vi "open camera settings.vi"(8 "error in (no error)":errorcluster, 11 "Camera Tester in":refnum<class "Camera Tester.lvclass">) -> (0 "error out":errorcluster, 3 "Camera Tester out":refnum<class "Camera Tester.lvclass">)   [LabVIEW 2014, in "Camera Tester.lvlib" / "Camera Tester.lvclass"]
uses:
  Camera Tester.lvclass
  Camera Tester.lvclass/Camera Tester.ctl
  <vilib>/ActorFramework/Message Enqueuer/Message Enqueuer.lvclass/Message Enqueuer.ctl
  <vilib>/ActorFramework/Message Enqueuer/Enqueue.vi
  <vilib>/ActorFramework/Message Priority Queue/Priority Enqueue.vi
  Camera Actor/Camera Actor Messages/open camera settings Msg/open camera settings Msg.lvclass
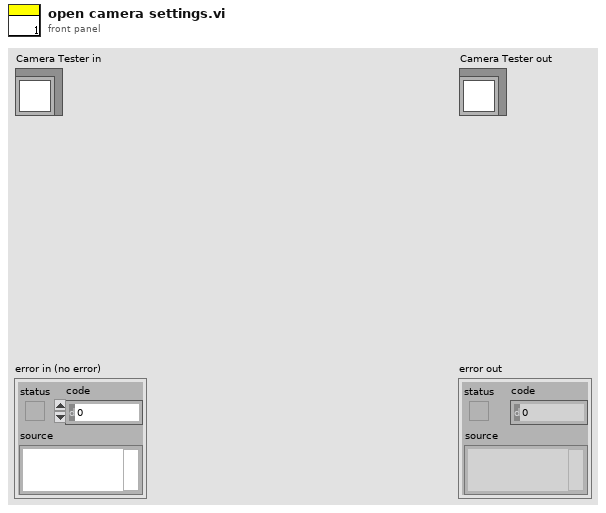
[diagram p1: front panel]
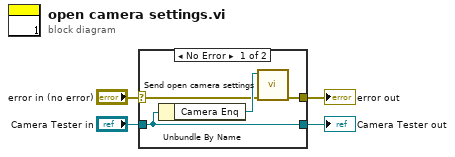
[diagram p0: block diagram]
diagram:
  n1 = case shown="No Error" "error in (no error)" {
    selector: "error in (no error)" -> [w6 w10]
    tunnel: [w5 w10] -> w3
    tunnel: [w8 w9] -> w1
    tunnel: "Camera Tester in" -> [w8 w9]
    frame No Error {
      n2 = Unbundle By Name(w8) -> ("Camera Enq"=w7:refnum<class "Message Enqueuer.lvclass">)
      n3 = call "Send open camera settings.vi"("error in (no error)"=w6, "Message Enqueuer"=w7) -> ("error out"=w5:errorcluster)  [unwired: 8 in, 1 out]
    }
    frame Error {
    }
  }
  "error out" <- w3
  "Camera Tester out" <- w1
